vi "MB Serial Slave Init.vi"(10 "Serial Port Setup (RT Only)":T1(array[cluster]) {"Termination Char" format="%.0x"; "Flow Control" items=["None"=0, "XON/XOFF"=1, "RTS/CTS"=2, "DTR/DSR"=4, "XON/XOFF & RTS/CTS"=3, "XON/XOFF & DTR/DSR"=5]; "Stop Bits" items=["1.0"=10, "1.5"=15, "2.0"=20]; "Data Bits" min=5 max=8 step=1}, 11 "VISA resource names":string[](array[string])) -> (1 "Any Errors":bool, 2 "All Errors":bool, 3 "VISA Sessions":refnum<visa-resource-name>[](array[refnum]))   [LabVIEW 2023, in "Voegtlin_NI_SMART_Modbus_Drivers.lvlib"]
uses:
  Voegtlin_NI_SMART_Modbus_Drivers.lvlib
  <vilib>/Instr/_visa.llb/VISA Open Access Mode.ctl
  <vilib>/Instr/_visa.llb/VISA Configure Serial Port (Instr).vi
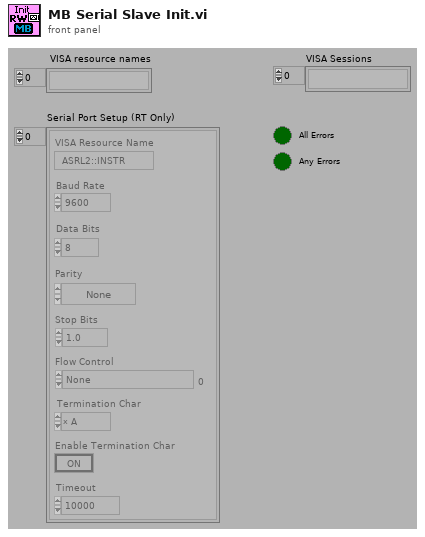
[diagram p1: front panel]
types:
  T1 = cluster{"VISA Resource Name":string, "Baud Rate":u32, "Data Bits":u16, "Parity":enum16{"None", "Odd", "Even", "Mark", "Space"}, "Stop Bits":u16, "Flow Control":u16, "Termination Char":u8, "Enable Termination Char":bool, "Timeout":u32}[]
  T2 = cluster{"VISA Resource Name":string, "Baud Rate":u32, "Data Bits":u16, "Parity":enum16{"None", "Odd", "Even", "Mark", "Space"}, "Stop Bits":u16, "Flow Control":u16, "Termination Char":u8, "Enable Termination Char":bool, "Timeout":u32}
  T3 = typedef "VISA Open Access Mode.ctl" = u32
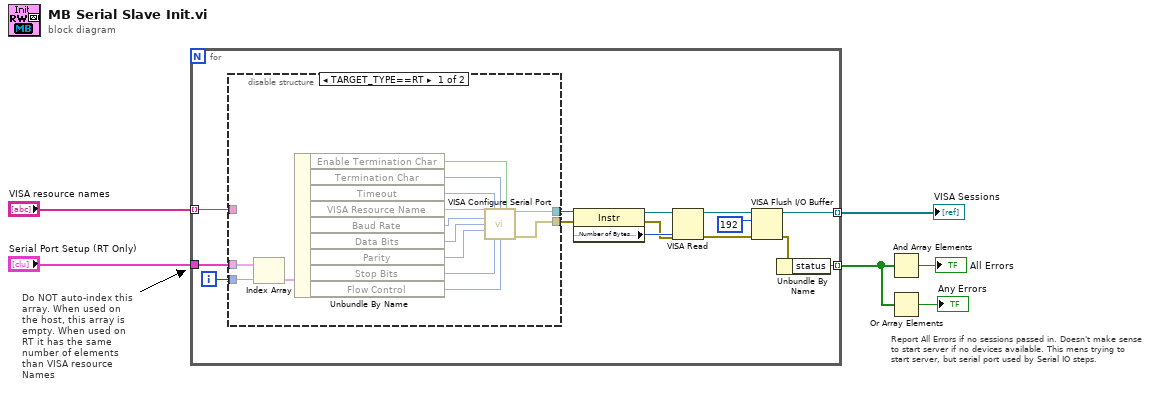
[diagram p0: block diagram]
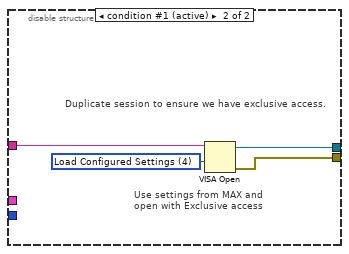
[diagram p2: hidden frame]
diagram:
  # "Report All Errors if no sessions passed in. Doesn't make sense to start server if no devices available. This mens trying to start server, but serial port used by Serial IO steps."
  # "Do NOT auto-index this array. When used on the host, this array is empty. When used on RT it has the same number of elements than VISA resource Names"
  n1 = for {
    tunnel: "VISA resource names" -> [w9] mode=indexing
    tunnel: [w12] -> w5 mode=indexing
    tunnel: "Serial Port Setup (RT Only)" -> [w11]
    tunnel: [w7] -> w4 mode=indexing
    i -> [w10]
    n2 = disable-structure shown="TARGET_TYPE==RT" {
      disable-tunnel: [w34 w37] -> w14
      disable-tunnel: [w33 w36] -> w13
      disable-tunnel: w11 -> [w32 _]
      disable-tunnel: w10 -> [w31 _]
      disable-tunnel: w9 -> [_ w38]
      frame condition #0 {
        n3 = Index Array(array=w32, index=w31) -> (element=w22:T2)
        n4 = Unbundle By Name(w22) -> ("Enable Termination Char"=w26:bool, "Termination Char"=w25:u8, "Timeout"=w27:u32, "VISA Resource Name"=w21:string, "Baud Rate"=w30:u32, "Data Bits"=w29:u16, "Parity"=w28:enum16{"None", "Odd", "Even", "Mark", "Space"}, "Stop Bits"=w24:u16, "Flow Control"=w23:u16)
        n5 = call-poly "VISA Configure Serial Port"("VISA resource name"=w21, "timeout (10sec)"=w27, "termination char\n(0xA = '\\n' = LF)"=w25, "Enable Termination\nChar (T)"=w26, "baud rate (9600)"=w30, "data bits (8)"=w29, "parity (0:none)"=w28, "stop bits (10: 1 bit)"=w24, "flow control (0:none)"=w23) -> ("VISA resource name out"=w34:refnum<visa-resource-name>, "error out"=w33:errorcluster)  [unwired: 5 in]
      }
      frame condition #1 (active) {
        w35 = T3 4 items=["VISA Defaults"=0, "Exclusive Lock"=1, "Load Configured Settings"=4] ("Access Mode")
        # "Duplicate session to ensure we have exclusive access."
        # "Use settings from MAX and open with Exclusive access"
        n6 = VISA Open(access mode=w35, VISA resource name=w38) -> (VISA resource name=w37:refnum<visa-resource-name>, error out=w36:errorcluster)  [unwired: 1 in, 2 out]
      }
    }
    n7 = property class="Instr"(reference=w14, error in=w13) -> (reference out=w20:refnum<visa-resource-name>, error out=w18:errorcluster, "Serial Settings:Number of Bytes at Serial Port"=w19:u32)
    n8 = VISA Read(VISA resource name=w20, byte count=w19, error in (no error)=w18) -> (VISA resource name out=w15:refnum<visa-resource-name>, error out=w16:errorcluster)  [unwired: 2 out]
    n9 = VISA Flush I/O Buffer(VISA resource name=w15, mask (16)=u16 192, error in (no error)=w16) -> (VISA resource name out=w12:refnum<visa-resource-name>, error out=w8:errorcluster)
    n10 = Unbundle By Name(w8) -> ("status"=w7:bool)
  }
  "VISA Sessions" <- w5
  n11 = And Array Elements(Boolean array=w4) -> (logical AND=→"All Errors":bool)
  n12 = Or Array Elements(Boolean array=w4) -> (logical OR=→"Any Errors":bool)
